vi "Set.vi"(7 "Description":string, 8 "Command Info In":T1, 10 "Setpoint (Top is = True )":bool) -> (0 "Command Info Out":T1)   [LabVIEW 2015]
uses:
  <vilib>/Rock Robotics/WPI/Framework/Command Status Info.ctl
  <vilib>/Rock Robotics/WPI/Framework/Completion Status.ctl
  <vilib>/Rock Robotics/WPI/Framework/Completion Notifier.ctl
  Implementation/CDF Mechanism Setpoints.ctl
  Implementation/CDF Mechanism Operations.ctl
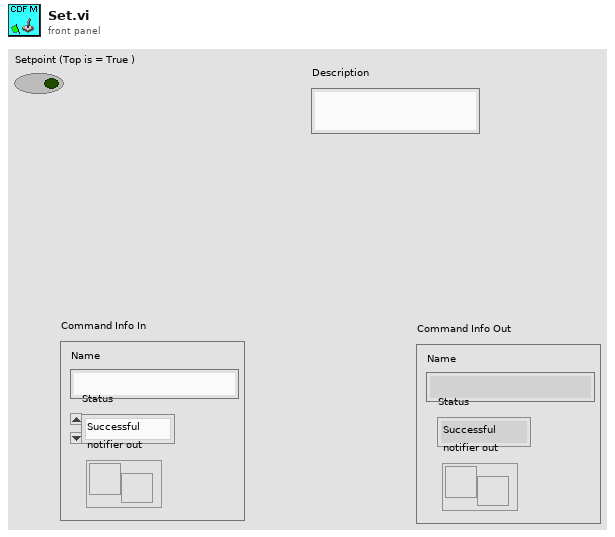
[diagram p1: front panel]
types:
  T1 = typedef "Command Status Info.ctl" = cluster{"Name":string, "Status":T2, "notifier out":T3}
  T2 = typedef "Completion Status.ctl" = enum16{"Successful", "Aborted", "Incomplete"}
  T3 = typedef "Completion Notifier.ctl" = refnum<notifier>
  T4 = typedef "CDF Mechanism Operations.ctl" = enum16{"Reserve", "Read Current", "Immediate", "Idle", "Flip", "Set", "Manual"}
  T5 = typedef "CDF Mechanism Setpoints.ctl" = cluster{"Operation":T4, "Setpoint":dbl, "Duration":dbl, "Setpoint (Top is = True )":bool}
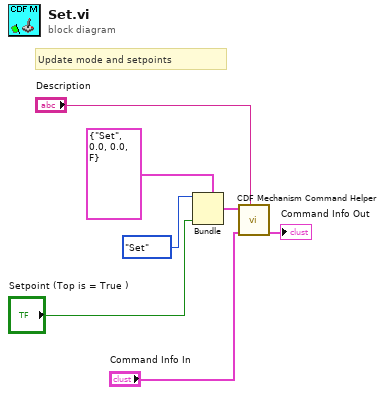
[diagram p0: block diagram]
diagram:
  # "Update mode and setpoints"
  n1 = Bundle(cluster=T5 {"Operation"=enum."Set", "Setpoint"=0.0, "Duration"=0.0, "Setpoint (Top is = True )"=FALSE} ("SubSystem Data"), "Operation"=CDF_Mechanism_Operations."Set", "Setpoint (Top is = True )"="Setpoint (Top is = True )") -> (w3:T5)  [unwired: 2 in]
  n2 = call "CDF Mechanism Command Helper.vi"("Description"="Description", "Command Info In"="Command Info In", "SubSystem Data"=w3) -> ("Command Info Out"=→"Command Info Out":T1)  [unwired: 7 in, 1 out]
